vi "mav_get.vi"(5 "stop":bool) -> (14 "HEARTBEAT #0":T3, 15 "ATTITUDE #30":T5, 16 "VFR_HUD #74":T4, 17 "GLOBAL_POSITION_INT #33":T2, 18 "STATUSTEXT":T1(array[cluster]))   [LabVIEW 2023]
uses:
  mav_global_var.vi
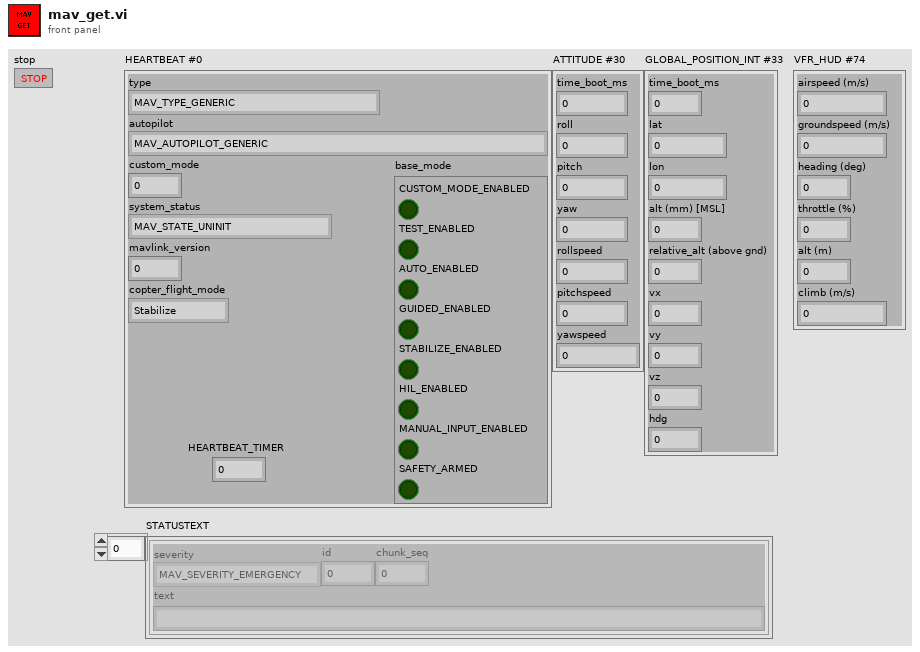
[diagram p1: front panel]
types:
  T1 = cluster{"severity":enum8{"MAV_SEVERITY_EMERGENCY", "MAV_SEVERITY_ALERT", "MAV_SEVERITY_CRITICAL", "MAV_SEVERITY_ERROR", "MAV_SEVERITY_WARNING", "MAV_SEVERITY_NOTICE", "MAV_SEVERITY_INFO", "MAV_SEVERITY_DEBUG"}, "id":u16, "chunk_seq":u8, "text":string}[]
  T2 = cluster{"time_boot_ms":u32, "lat":i32, "lon":i32, "alt (mm) [MSL]":i32, "relative_alt (above gnd)":i32, "vx":i16, "vy":i16, "vz":i16, "hdg":u16}
  T3 = cluster{"type":enum8{"MAV_TYPE_GENERIC", "MAV_TYPE_FIXED_WING", "MAV_TYPE_QUADROTOR", "MAV_TYPE_COAXIAL", "MAV_TYPE_HELICOPTER", "MAV_TYPE_ANTENNA_TRACKER", "MAV_TYPE_GCS", "MAV_TYPE_AIRSHIP", "MAV_TYPE_FREE_BALLOON", "MAV_TYPE_ROCKET", "MAV_TYPE_GROUND_ROVER", "MAV_TYPE_SURFACE_BOAT", "MAV_TYPE_SUBMARINE", "MAV_TYPE_HEXAROTOR", "MAV_TYPE_OCTOROTOR", "MAV_TYPE_TRICOPTER", "MAV_TYPE_FLAPPING_WING", "MAV_TYPE_KITE", "MAV_TYPE_ONBOARD_CONTROLLER", "MAV_TYPE_VTOL_TAILSITTER_DUOROTOR", "MAV_TYPE_VTOL_TAILSITTER_QUADROTOR", "MAV_TYPE_VTOL_TILTROTOR", "MAV_TYPE_VTOL_FIXEDROTOR", "MAV_TYPE_VTOL_TAILSITTER", "MAV_TYPE_VTOL_TILTWING", "MAV_TYPE_VTOL_RESERVED5", "MAV_TYPE_GIMBAL", "MAV_TYPE_ADSB", "MAV_TYPE_PARAFOIL", "MAV_TYPE_DODECAROTOR", "MAV_TYPE_CAMERA", "MAV_TYPE_CHARGING_STATION", "MAV_TYPE_FLARM", "MAV_TYPE_SERVO", "MAV_TYPE_ODID", "MAV_TYPE_DECAROTOR", "MAV_TYPE_BATTERY", "MAV_TYPE_PARACHUTE", "MAV_TYPE_LOG", "MAV_TYPE_OSD", "MAV_TYPE_IMU", "MAV_TYPE_GPS", "MAV_TYPE_WINCH", "MAV_TYPE_GENERIC_MULTIROTOR", "MAV_TYPE_ILLUMINATOR"}, "autopilot":enum8{"MAV_AUTOPILOT_GENERIC", "MAV_AUTOPILOT_RESERVED", "MAV_AUTOPILOT_SLUGS", "MAV_AUTOPILOT_ARDUPILOTMEGA", "MAV_AUTOPILOT_OPENPILOT", "MAV_AUTOPILOT_GENERIC_WAYPOINTS_ONLY", "MAV_AUTOPILOT_GENERIC_WAYPOINTS_AND_SIMPLE_NAVIGATION_ONLY", "MAV_AUTOPILOT_GENERIC_MISSION_FULL", "MAV_AUTOPILOT_INVALID", "MAV_AUTOPILOT_PPZ", "MAV_AUTOPILOT_UDB", "MAV_AUTOPILOT_FP", "MAV_AUTOPILOT_PX4", "MAV_AUTOPILOT_SMACCMPILOT", "MAV_AUTOPILOT_AUTOQUAD", "MAV_AUTOPILOT_ARMAZILA", "MAV_AUTOPILOT_AEROB", "MAV_AUTOPILOT_ASLUAV", "MAV_AUTOPILOT_SMARTAP", "MAV_AUTOPILOT_AIRRAILS", "MAV_AUTOPILOT_REFLEX"}, "custom_mode":u32, "system_status":enum16{"MAV_STATE_UNINIT", "MAV_STATE_BOOT", "MAV_STATE_CALIBRATING", "MAV_STATE_STANDBY", "MAV_STATE_ACTIVE", "MAV_STATE_CRITICAL", "MAV_STATE_EMERGENCY", "MAV_STATE_POWEROFF", "MAV_STATE_FLIGHT_TERMINATION"}, "mavlink_version":u8, "base_mode":cluster{"CUSTOM_MODE_ENABLED":bool, "TEST_ENABLED":bool, "AUTO_ENABLED":bool, "GUIDED_ENABLED":bool, "STABILIZE_ENABLED":bool, "HIL_ENABLED":bool, "MANUAL_INPUT_ENABLED":bool, "SAFETY_ARMED":bool}, "HEARTBEAT_TIMER":u32, "copter_flight_mode":enum32{"Stabilize", "Acro", "AltHold", "Auto", "Guided", "Loiter", "RTL", "Circle", "--Deprecated-8", "Land", "--Deprecated-10", "Drift", "--Deprecated-12", "Sport", "Flip", "AutoTune", "PosHold", "Brake", "Throw", "Avoid_ADSB", "Guided_NoGPS", "Smart_RTL", "FlowHold", "Follow", "ZigZag", "SystemID", "Heli_Autorotate", "Auto RTL"}}
  T4 = cluster{"airspeed (m/s)":sgl, "groundspeed (m/s)":sgl, "heading (deg) ":i16, "throttle (%) ":u16, "alt (m)":sgl, "climb (m/s)":sgl}
  T5 = cluster{"time_boot_ms":u32, "roll":sgl, "pitch":sgl, "yaw":sgl, "rollspeed":sgl, "pitchspeed":sgl, "yawspeed":sgl}
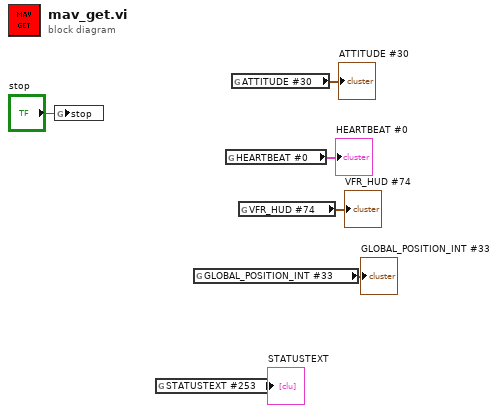
[diagram p0: block diagram]
diagram:
  n1 = global write "mav_global_var.vi" "stop"("stop") -> ()
  n2 = global read "mav_global_var.vi" "STATUSTEXT #253"() -> (→"STATUSTEXT":T1)
  n3 = global read "mav_global_var.vi" "GLOBAL_POSITION_INT #33"() -> (→"GLOBAL_POSITION_INT #33":T2)
  n4 = global read "mav_global_var.vi" "HEARTBEAT #0"() -> (→"HEARTBEAT #0":T3)
  n5 = global read "mav_global_var.vi" "ATTITUDE #30"() -> (→"ATTITUDE #30":T5)
  n6 = global read "mav_global_var.vi" "VFR_HUD #74"() -> (→"VFR_HUD #74":T4)
